vi "Send UI Reference.vi"(8 "error in (no error)":errorcluster, 11 "Camera Prime95B Controller in":refnum<class "Camera Prime95B Controller.lvclass">) -> (0 "error out":errorcluster, 3 "Camera Prime95B Controller out":refnum<class "Camera Prime95B Controller.lvclass">)   [LabVIEW 2020, in "Camera_Prime95B.lvlib" / "Camera Prime95B Controller.lvlib" / "Camera Prime95B Controller.lvclass"]
uses:
  Camera Prime95B Controller.lvclass
  C:/Program Files/National Instruments/LabVIEW 2020/vi.lib/ActorFramework/Actor/Actor.lvclass
  <vilib>/ActorFramework/Actor/Actor.lvclass/Actor.ctl
  Camera Prime95B Controller.lvclass/Camera Prime95B Controller.ctl
  HAL Layer/Component/Device/Device Messages/SendPanelUIReference Msg/SendPanelUIReference Msg.lvclass/SendPanelUIReference Msg.ctl
  <vilib>/ActorFramework/Message Enqueuer/Message Enqueuer.lvclass/Message Enqueuer.ctl
  <vilib>/ActorFramework/Message Enqueuer/Enqueue.vi
  HAL Layer/Component/Device/Device Messages/SendPanelUIReference Msg/SendPanelUIReference Msg.lvclass
  C:/Program Files/National Instruments/LabVIEW 2020/vi.lib/ActorFramework/Message/Message.lvclass
  <vilib>/ActorFramework/Message Priority Queue/Priority Enqueue.vi
  <vilib>/ActorFramework/Actor/Actor.lvclass
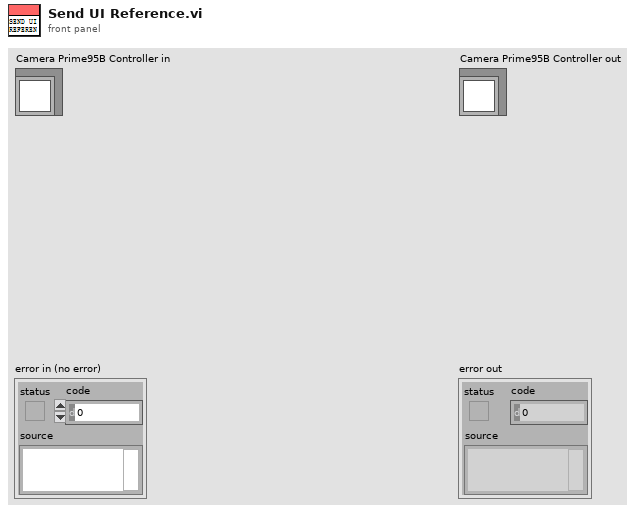
[diagram p1: front panel]
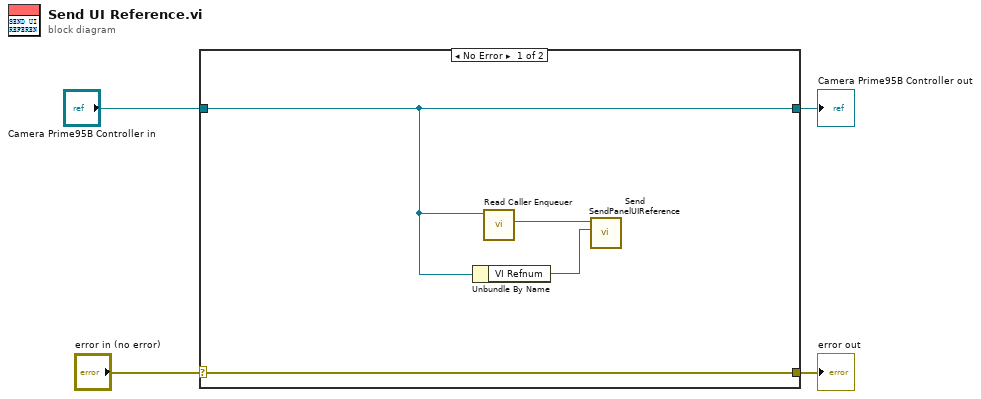
[diagram p0: block diagram]
diagram:
  n1 = case shown="No Error" "error in (no error)" {
    selector: "error in (no error)" -> [w8 w10]
    tunnel: [w8 w10] -> w3
    tunnel: [w5 w9] -> w1
    tunnel: "Camera Prime95B Controller in" -> [w5 w9]
    frame No Error {
      n2 = Unbundle By Name(w5) -> ("VI Refnum"=w6:refnum<vi>)
      n3 = call <vilib>:"Read Caller Enqueuer.vi"("Actor"=w5) -> ("Caller Enqueuer"=w7:refnum<class "Message Enqueuer.lvclass">)  [unwired: 10 in]
      n4 = call "Send SendPanelUIReference.vi"("VI Refnum"=w6, "Message Enqueuer"=w7) -> ()  [unwired: 8 in, 2 out]
    }
    frame Error {
    }
  }
  "error out" <- w3
  "Camera Prime95B Controller out" <- w1
